vi "iTC Tests.vi"() -> ()   [LabVIEW 2014]
uses:
  <instrlib>/Mercury iXX/Public/Libraries/System/Open/Open System.vi
  <instrlib>/Mercury iXX/Public/Libraries/Temperature/Open/Open Temperature Device.vi
  <instrlib>/Mercury iXX/Public/Libraries/Temperature/Signals/Read/Temperature (Read).vi
  <instrlib>/Mercury iXX/Mercury iXX.lvlib
  <instrlib>/Mercury iXX/Public/Libraries/System.lvlib
  <instrlib>/Mercury iXX/Public/Libraries/Temperature.lvlib
panel:
  in  "Stop":bool
  out "AB1":dbl
  out "Error Text":string
  out "Error #":dbl
  out "Error":bool
  out "CCS":dbl
  in  "VISA resource name":refnum<visa-resource-name>="MERCURYITC"
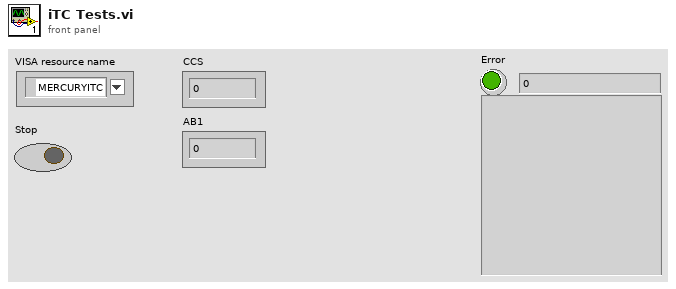
[diagram p1: front panel]
types:
  T1 = typedef "Mercury iXX.lvlib/Mercury Reference.ctl" = cluster{"Comms":refnum<visa-resource-name>, "Device ID":string[], "Comms Layer":T2, "Command":string, "Query reference":T3}
  T2 = typedef "Mercury iXX.lvlib/Comms Transport Layer.ctl" = enum16{"Ethernet TCP/IP", "USB", "ISOBus - RS-232", "GPIB"}
  T3 = typedef "Mercury iXX.lvlib/Query Dynamic Reference.ctl" = refnum<vi>
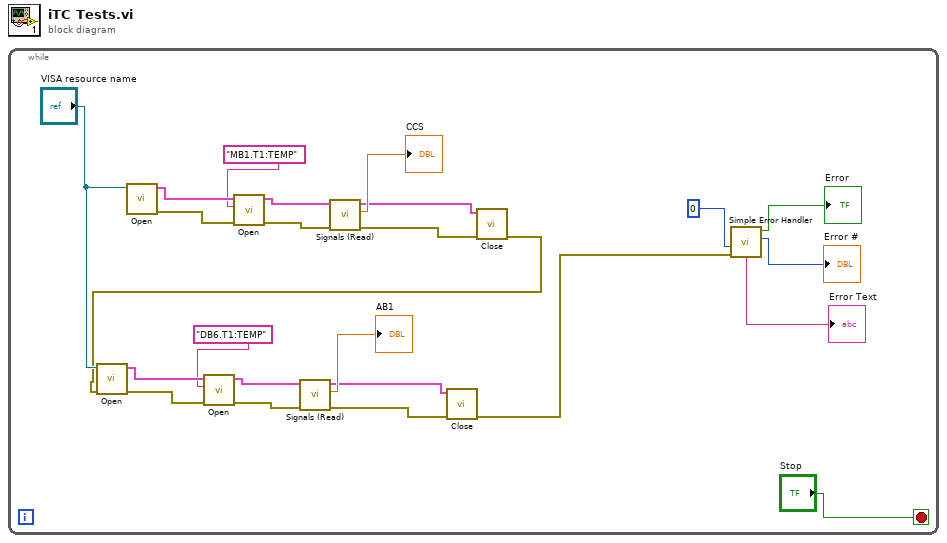
[diagram p0: block diagram]
diagram:
  n1 = while {
    stop <- "Stop" stop-if-true
    n2 = call-poly <instrlib>:"Open.vi"("VISA resource name"="VISA resource name") -> ("error out"=w22:errorcluster, "Mercury Reference Out"=w24:T1)  [unwired: 6 in, 3 out]
    n3 = call-poly <instrlib>:"Open.vi"("error in (no error)"=w22, "Device Identifier"="MB1.T1:TEMP", "Mercury Reference In"=w24) -> ("error out"=w19:errorcluster, "Mercury Reference Out"=w21:T1)  [unwired: 7 in]
    n4 = call-poly <instrlib>:"Signals (Read).vi"("error in"=w19, "Mercury Reference In"=w21) -> ("error out"=w14:errorcluster, "Temperature"=→"CCS":dbl, "Mercury Reference Out"=w13:T1)  [unwired: 5 in, 2 out]
    n5 = call <instrlib>:"Close.vi"("error in (no error)"=w14, "Mercury Reference"=w13) -> ("error out"=w3:errorcluster)  [unwired: 9 in]
    n6 = call-poly <instrlib>:"Open.vi"("error in (no error)"=w3, "VISA resource name"="VISA resource name") -> ("error out"=w10:errorcluster, "Mercury Reference Out"=w12:T1)  [unwired: 5 in, 3 out]
    n7 = call-poly <instrlib>:"Open.vi"("error in (no error)"=w10, "Device Identifier"="DB6.T1:TEMP", "Mercury Reference In"=w12) -> ("error out"=w7:errorcluster, "Mercury Reference Out"=w9:T1)  [unwired: 7 in]
    n8 = call-poly <instrlib>:"Signals (Read).vi"("error in"=w7, "Mercury Reference In"=w9) -> ("error out"=w6:errorcluster, "Temperature"=→"AB1":dbl, "Mercury Reference Out"=w5:T1)  [unwired: 5 in, 2 out]
    n9 = call <instrlib>:"Close.vi"("error in (no error)"=w6, "Mercury Reference"=w5) -> ("error out"=w2:errorcluster)  [unwired: 9 in]
    n10 = call <vilib>:"Simple Error Handler.vi"("type of dialog (OK msg:1)"=0, "error in (no error)"=w2) -> ("error?"=→"Error":bool, "code out"=→"Error #":i32, "message"=→"Error Text":string)  [unwired: 3 in, 2 out]
  }
